vi "Configure Input Attenuation.vi"(0 "VISA resource name":refnum<visa-resource-name>, 5 "Platform Slot Number (10)":i16=10 min=-1 max=255, 7 "Input Attenuation (0:MINimum)":i32(ring) items=["MINimum", "MAXimum", "DEFault", "User Defined Value"], 9 "User Defined Attenuation Value (5.0000)":dbl=5.0 format="%_5g", 11 "error in (no error)":errorcluster) -> (4 "VISA resource name out":refnum<visa-resource-name>, 15 "error out":errorcluster)   [LabVIEW 2018, in "LTB-1.lvlib" / "3150.lvlib"]
doc: "Configures the absolute attenuation, in dB, to a specific value. The valid range of values depends on the type of instrument and the current wavelength. This value is used only when the ATTenuation control mode is active."
uses:
  3150.lvlib
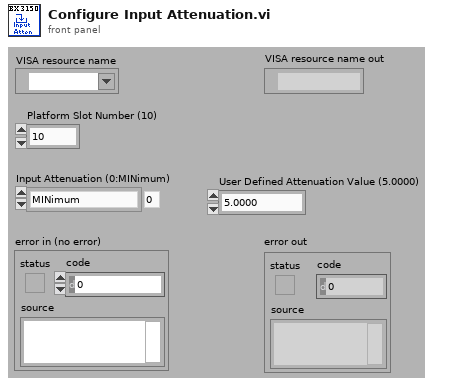
[diagram p1: front panel]
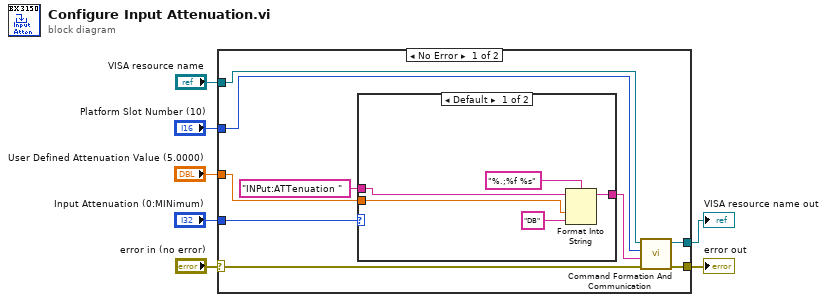
[diagram p0: block diagram]
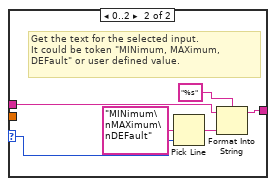
[diagram p2: hidden frame]
diagram:
  n1 = case shown="No Error" "error in (no error)" {
    selector: "error in (no error)" -> [w11 w29]
    tunnel: "VISA resource name" -> [w13 w28]
    tunnel: [w9 w29] -> w5
    tunnel: "Input Attenuation (0:MINimum)" -> [w16 _]
    tunnel: "Platform Slot Number (10)" -> [w12 _]
    tunnel: [w10 w28] -> w2
    tunnel: "User Defined Attenuation Value (5.0000)" -> [w8 _]
    frame No Error {
      n2 = case shown="Default" w16 {
        selector: w16 -> [_ w23]
        tunnel: "INPut:ATTenuation " ("Command") -> [w19 w24]
        tunnel: [w20 w22] -> w14
        tunnel: w8 -> [w18 _]
        frame Default {
          n3 = Format Into String(format string="%.;%f %s", initial string=w19, w18, "DB" ("multi-line string")) -> (resulting string=w20:string)  [unwired: 1 in, 1 out]
        }
        frame 0..2 {
          # "Get the text for the selected input.\nIt could be token \"MINimum, MAXimum,\nDEFault\" or user defined value."
          n4 = Pick Line(multi-line string="MINimum\nMAXimum\nDEFault", line index=w23) -> (output string=w25:string)  [unwired: 1 out]
          n5 = Format Into String(format string="%s", initial string=w24, w25) -> (resulting string=w22:string)  [unwired: 1 in, 1 out]
        }
      }
      n6 = call "Command Formation And Communication.vi"("error in (no error)"=w11, "Command"=w14, "Platform Slot Number"=w12, "VISA resource name"=w13) -> ("error out"=w9:errorcluster, "VISA resource name out"=w10:refnum<visa-resource-name>)  [unwired: 1 in, 5 out]
    }
    frame Error {
    }
  }
  "VISA resource name out" <- w2
  "error out" <- w5
